vi "XIPIN_Video_Direct_Memory_Access_1_1.vi"   [LabVIEW 2017]
doc: "The Xilinx Video DMA LogiCORE provides a flexible interface for controlling and synchronizing video frame stores from external memory. The VDMA works in conjunction with the Video Frame Buffer Controller (VFBC) and provides a read or a write interface to external memory. Multiple VDMAs from different clock domains can be linked together to control frame store reads and writes from multiple sources. Automatic frame skips and repeats are performed to seamlessly allow frame rate conversion. Support for up to 16 external frame stores with image sizes of 4k x 4k is provided. The core is programmable through a comprehensive register interface for setting and controlling frame synchronization (can be turned on/off in real-time), frame read/write delays, source synchronization switching, circular buffer enable and more using logic or a microprocessor. A comprehensive set of interrupt status bits provided for processor monitoring. The LogiCORE is provided with two different interfaces: General Purpose Processor and EDK pCore (including device driver).\n------------------------------------\n<b>Need License</b> : Yes"
uses:
  <vilib>/rvi/XilinxIP/XIPIN_XNode/niFpgaXIPIN.xnode
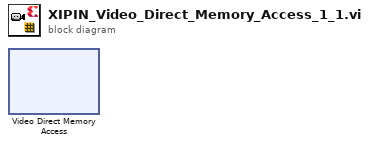
[diagram p0: block diagram]
diagram:
  n1 = xnode ("Video Direct Memory Access")() -> ()
